vi "Sinc generator to TDMS.vi"() -> ()   [LabVIEW 2025]
uses:
  <vilib>/Analysis/1siggen.llb/Ramp Pattern by Samples.vi
  <vilib>/Analysis/4window.llb/Hamming Window (DBL).vi
  <vilib>/Analysis/2dsp.llb/Real FFT.vi
  <vilib>/Analysis/4window.llb/AllCosWindow (DBL).vi
  <vilib>/Analysis/NI_AALBase.lvlib
  <vilib>/Analysis/NI_AALPro.lvlib
panel:
  in  "Settings Tabs":T1(tab)
  in  "fc":dbl=567000.0 format="%#_6p"
  in  "Tp":dbl=0.0001 format="%#_6p"
  in  "TBW":dbl=4.0
  in  "Vpk":dbl=0.05 format="%#_6p"
  out "BW":dbl
  out "dt/Ts":dbl
  out "N":dbl
  out "Start":dbl format="%#_6p"
  out "End":dbl format="%#_6p"
  out "fs":dbl format="%#_6p"
  out "RF Size":i32
  out "1/fs":dbl format="%#_6p"
  in  "Delays":T2={"gate_delay"=1e-05, "damping_delay"=5e-06, "initial_delay"=5e-06, "final_delay"=5e-06} {"initial_delay" format="%#_6ps"; "final_delay" format="%#_6ps"; "gate_delay" format="%#_6ps"; "damping_delay" format="%#_6ps"}
  in  "Vhigh":dbl=5.0
  out "Gate Delay Size":i32
  out "Damping Delay Size":i32
  out "Initial Delay Size":i32
  out "Final Delay Size":i32
  in  "Digital Wfm Resampling":enum32{"Same Fs As RF Wfm", "Resampled Fs"}(tab)
  out "Digital Wfm Fs":dbl format="%#_6p"
  out "Digital Wfm dt":dbl format="%#_6p"
  in  "Digital Wfm Resampled Fs":dbl=300000.0 format="%#_6p"
  in  "Wfm Group Name Suffix":string="Wfm1"
  in  "TDMS File Path":path
  in  "Results Tab":T3(tab)
  out "sinc pluse":waveform(dbl)(graph)
  out "carrier":waveform(dbl)(graph)
  out "RF sinc pluse":waveform(dbl)(graph)
  out "RF Pulse Spectrrum Graph":cluster{"Ramp Pattern":dbl[], dbl[]}(graph)
  out "Gate IN":waveform(dbl)(graph)
  out "Damping":waveform(dbl)(graph)
  out "Rx ON":waveform(dbl)(graph)
  out "Modulated RF Signal":waveform(dbl)(graph)
  out "PA ON":waveform(dbl)(graph)
  # "Carrier Frequency fc = 567 kHz\n  - Sampling Frequency fs = 20 x fc\nPluse Duration Tp = 100 us\nTime Bandwidth Product TBW = 4\n  - Bandwidth BW = TBW/Tp\nPeak Amplitude Vpk = 50 mV"
  # "If TDMS File Path specified,\nwill create/replace file"
  # "Example:\nIf Wfm Group Name Suffix = Wfm1, then it creates:\n- FGEN_Wfm1\n    - Chn0\n- DAQ_Wfm1\n    - PA ON\n    - Gate IN\n    - Damping \n    - Rx ON"
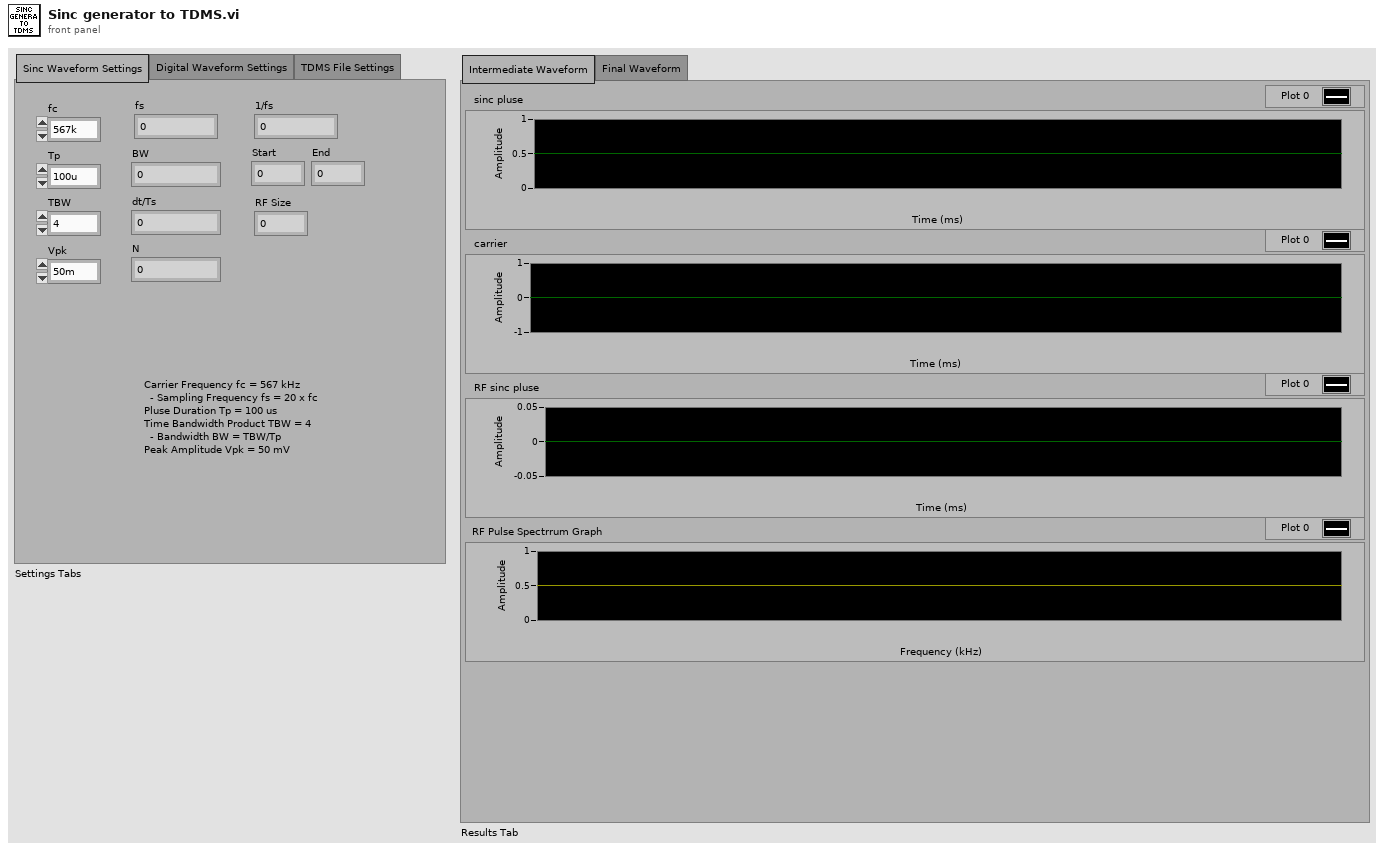
[diagram p1: front panel]
types:
  T1 = enum32{"Sinc Waveform Settings", "Digital Waveform Settings", "TDMS File Settings"}
  T2 = cluster{"gate_delay":dbl, "damping_delay":dbl, "initial_delay":dbl, "final_delay":dbl}
  T3 = enum32{"Intermediate Waveform", "Final Waveform"}
  T4 = enum16{"open", "open or create", "create or replace", "create", "open (read-only)"}
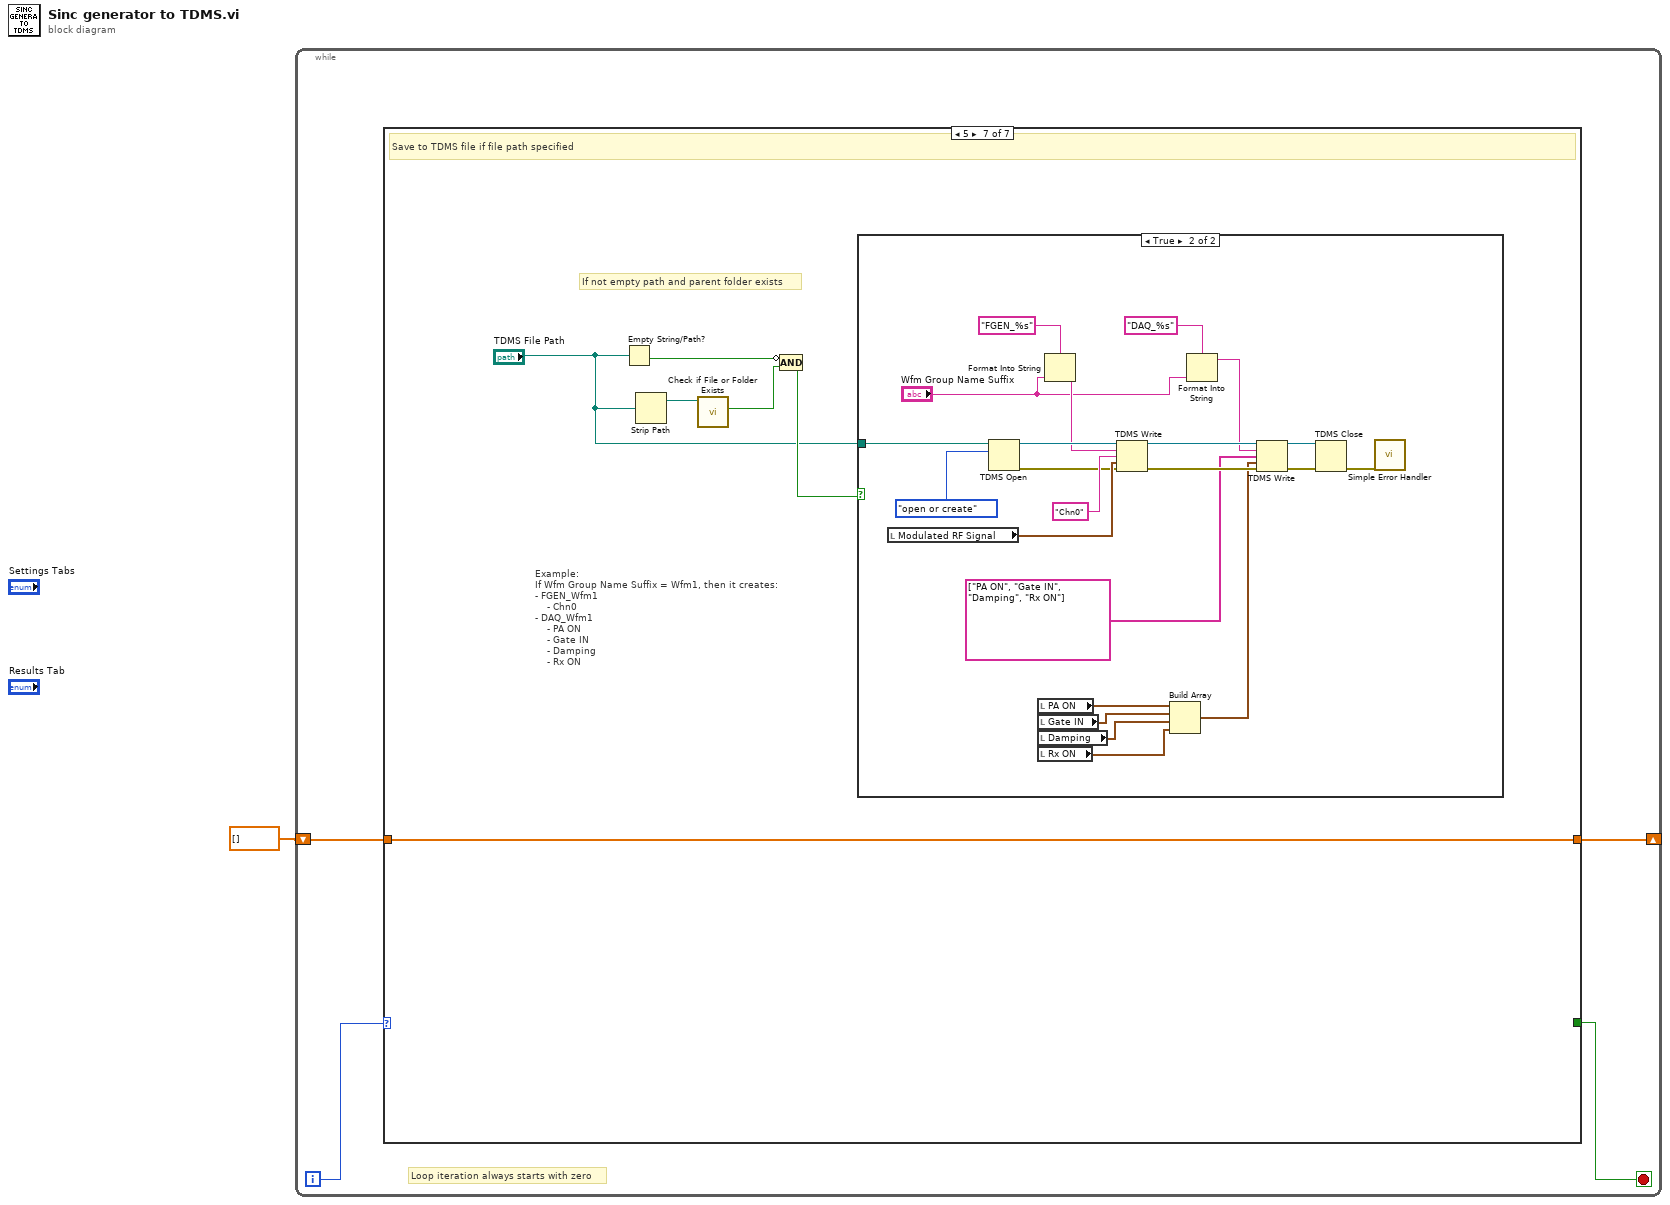
[diagram p0: block diagram]
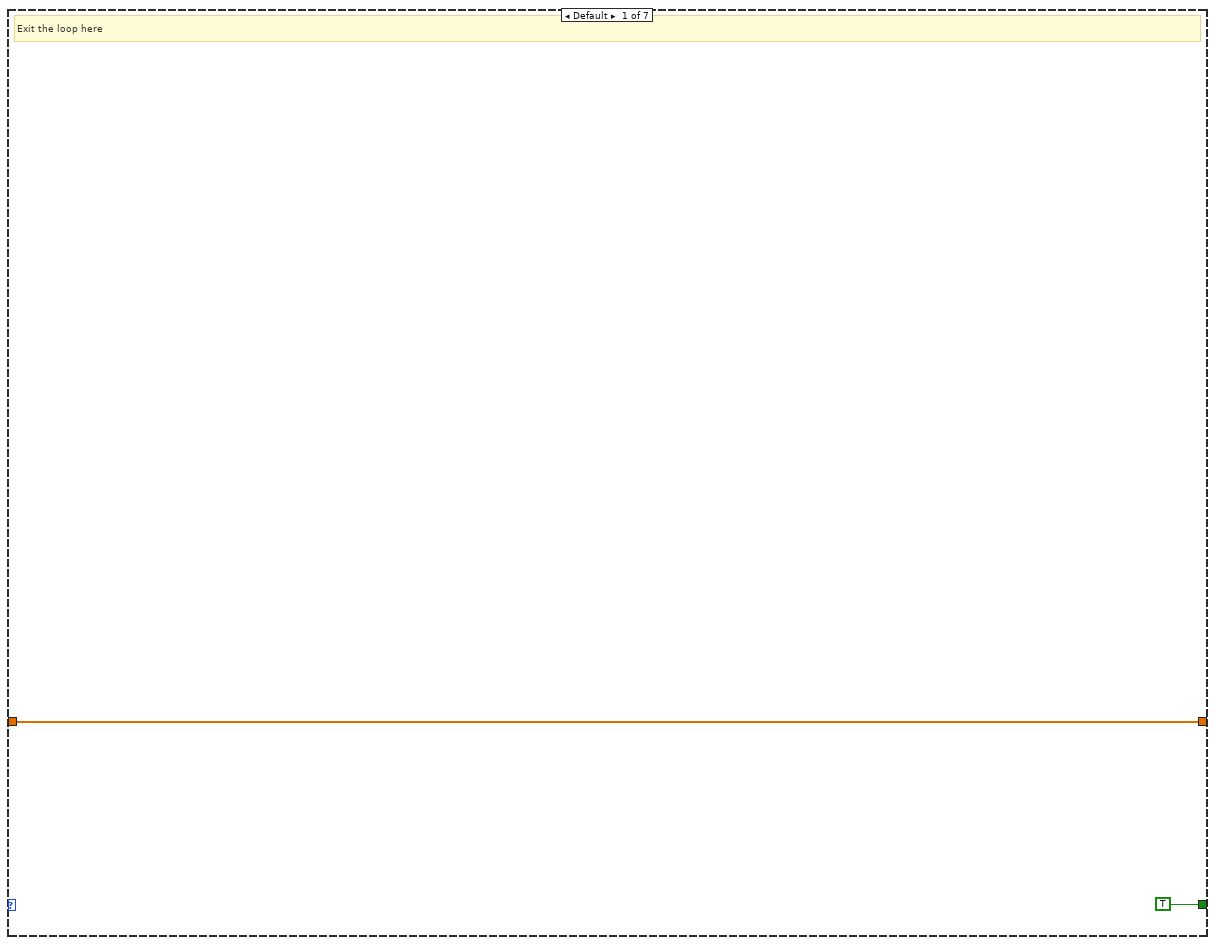
[diagram p2: hidden frame]
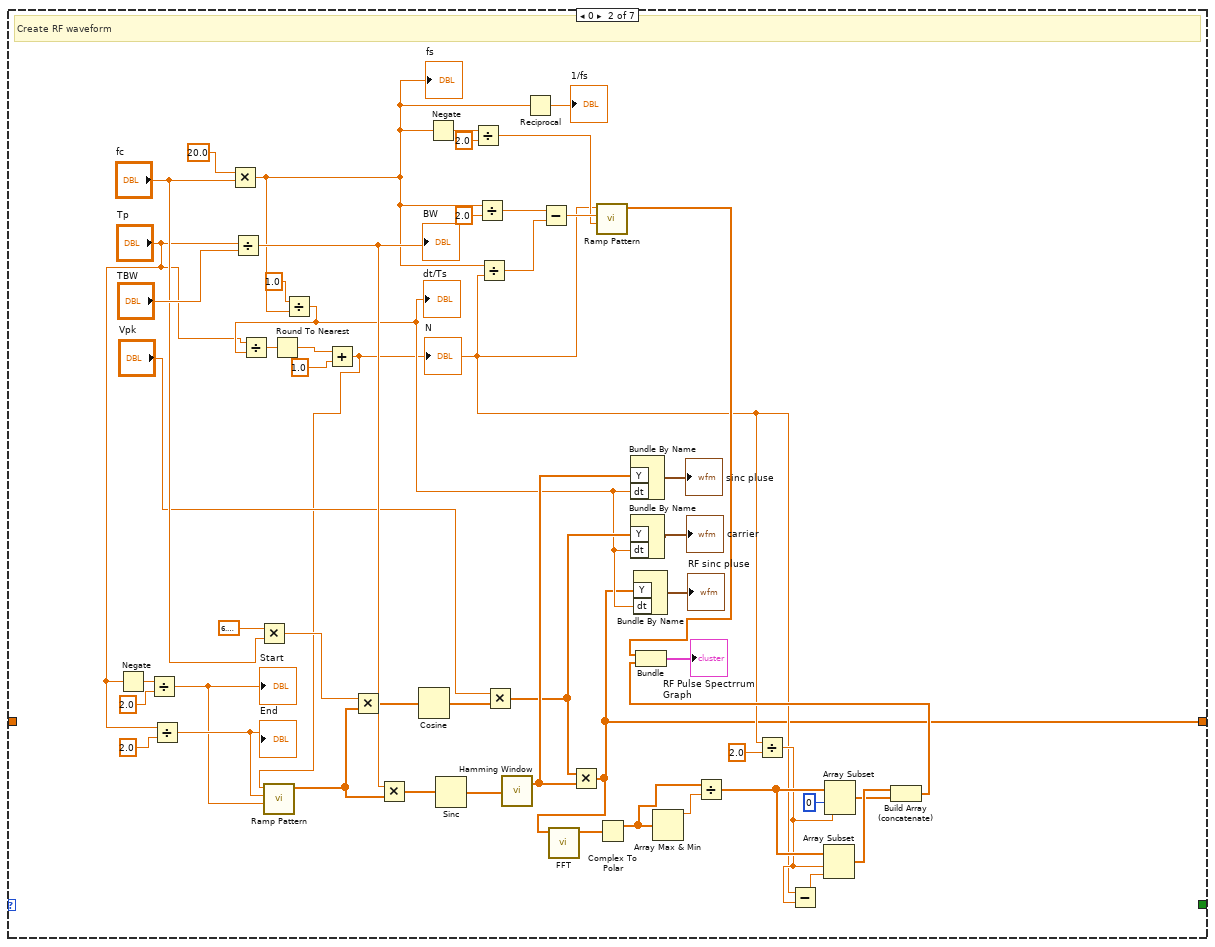
[diagram p3: hidden frame]
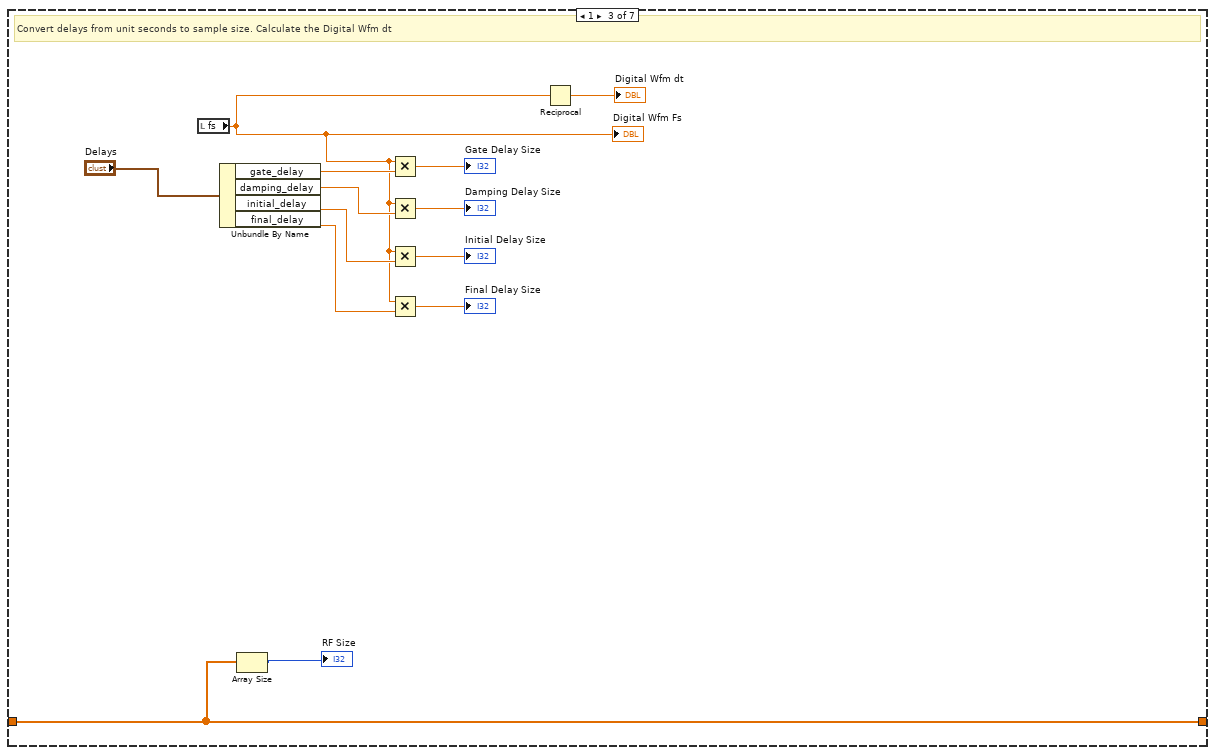
[diagram p4: hidden frame]
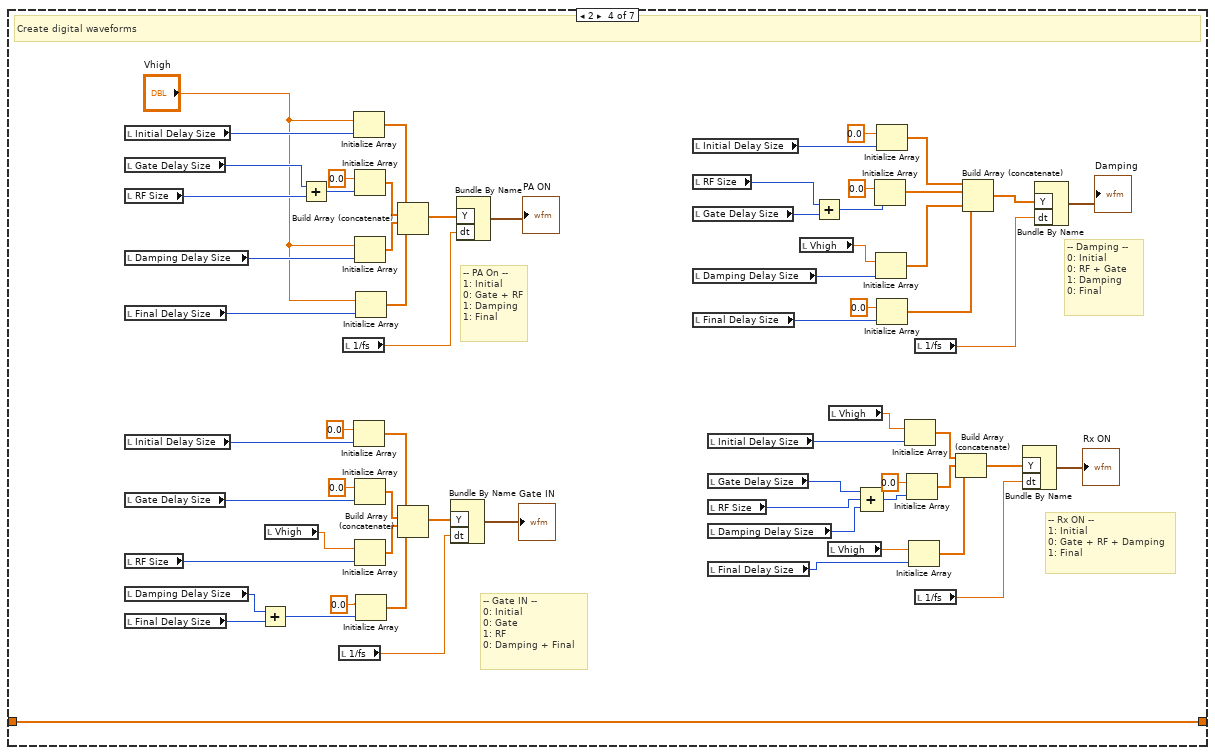
[diagram p5: hidden frame]
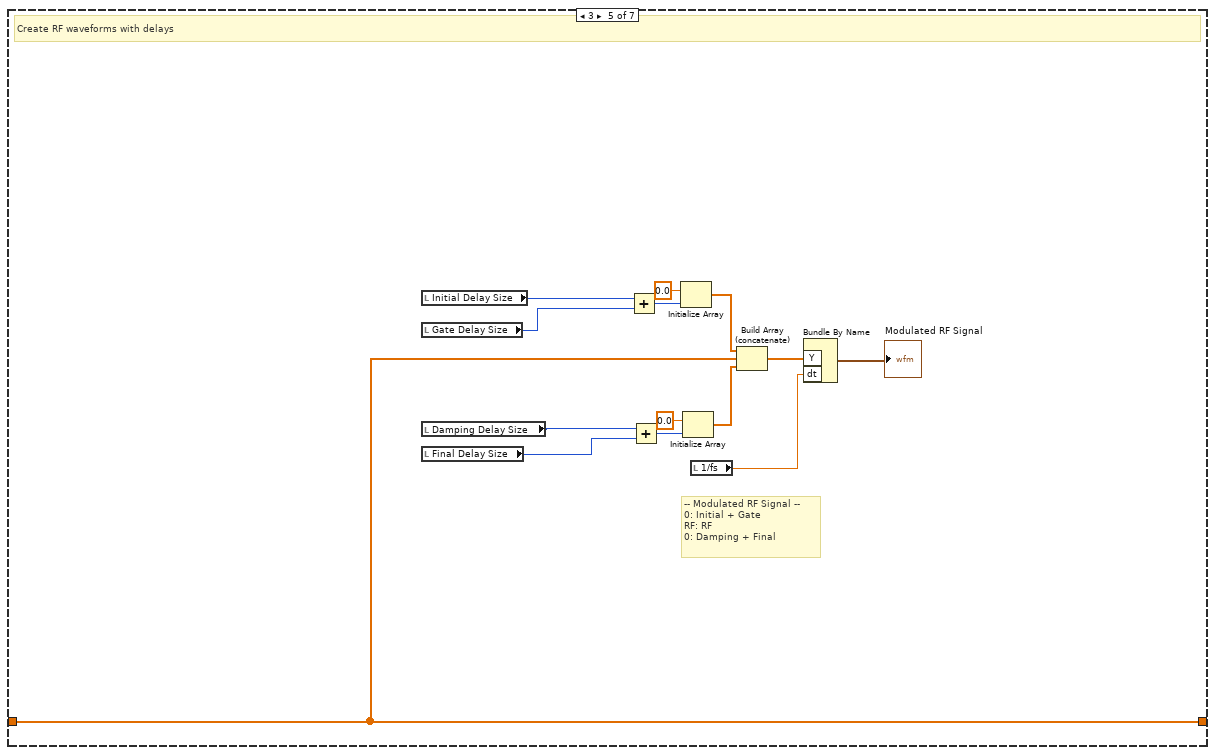
[diagram p6: hidden frame]
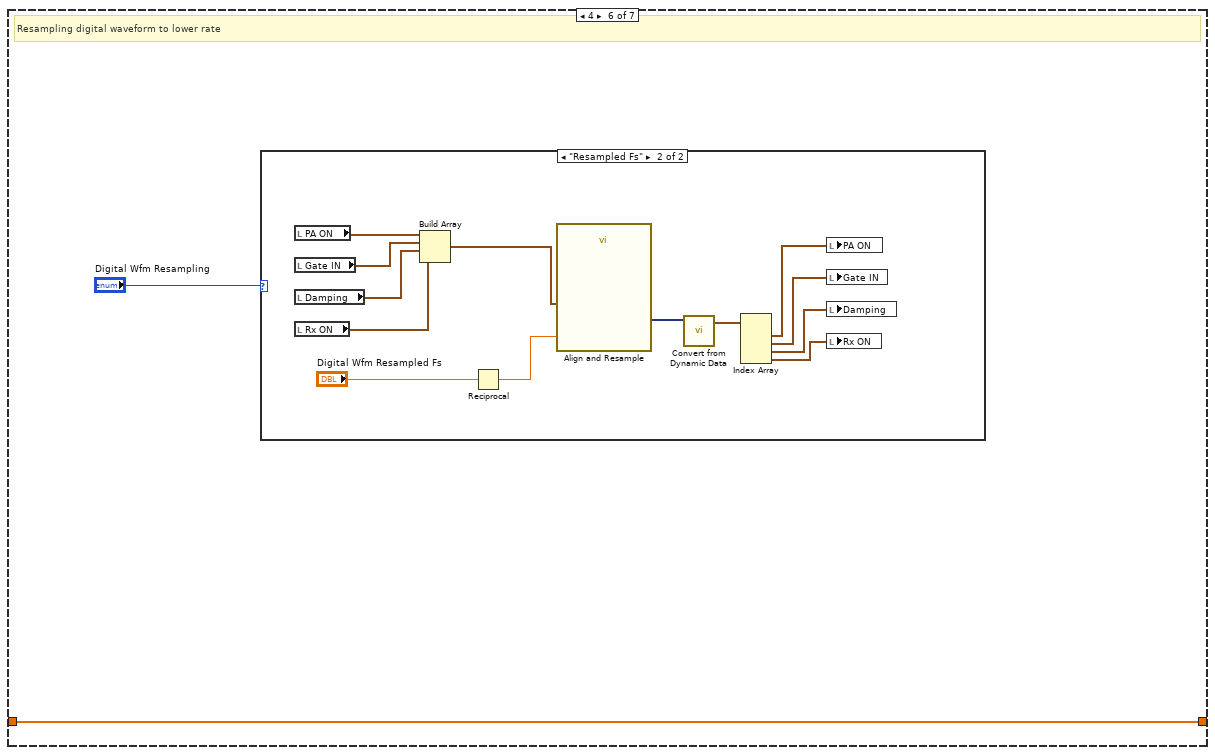
[diagram p7: hidden frame]
diagram:
  n1 = while {
    shift-right: [w4] -> _
    shift-left: dbl[] [] -> [w3]
    i -> [w5]
    stop <- w2 stop-if-true
    # "Loop iteration always starts with zero"
    n2 = case shown="5" w5 {
      tunnel: [TRUE _ _ _ _ _ _] -> w2
      tunnel: [w6 w10 w64 w137 w142 w153 w172] -> w4
      tunnel: w3 -> [w6 _ w64 w137 w142 w153 w172]
      frame Default {
        # "Exit the loop here"
      }
      frame 0 {
        # "Create RF waveform"
        n3 = Negate(x="Tp") -> (-x=w21:dbl)
        n4 = Divide(x=w21, y=2.0) -> (x/y=w32:dbl)
        "Start" <- w32
        n5 = Divide(x="Tp", y=2.0) -> (x/y=w51:dbl)
        "End" <- w51
        n6 = Multiply(x=20.0, y="fc") -> (x*y=w8:dbl)
        "fs" <- w8
        n7 = Divide(x="TBW", y="Tp") -> (x/y=w49:dbl)
        "BW" <- w49
        n8 = Multiply(x=6.283185307179586, y="fc") -> (x*y=w45:dbl)
        n9 = Divide(x=1.0, y=w8) -> (x/y=w22:dbl)
        "dt/Ts" <- w22
        n10 = Divide(x="Tp", y=w22) -> (x/y=w54:dbl)
        n11 = Round To Nearest(number=w54) -> (nearest integer value=w56:dbl)
        n12 = Add(x=w56, y=1.0) -> (x+y=w11:dbl)
        "N" <- w11
        n13 = call-poly <vilib>:"Ramp Pattern.vi"("start"=w32, "end"=w51, "samples"=w11) -> ("Ramp Pattern"=w23:dbl[])  [unwired: 7 in, 1 out]
        n14 = Multiply(x=w45, y=w23) -> (x*y=w44:dbl[])
        n15 = Multiply(x=w49, y=w23) -> (x*y=w50:dbl[])
        n16 = Cosine(x=w44) -> (cos(x)=w42:dbl[])
        n17 = Negate(x=w8) -> (-x=w19:dbl)
        n18 = Sinc(1:w50) -> (0:w48:dbl[])
        n19 = Divide(x=w19, y=2.0) -> (x/y=w13:dbl)
        n20 = Divide(x=w8, y=2.0) -> (x/y=w16:dbl)
        n21 = Divide(x=w8, y=w11) -> (x/y=w15:dbl)
        n22 = Multiply(x="Vpk", y=w42) -> (x*y=w29:dbl[])
        n23 = call-poly <vilib>:"Hamming Window.vi"("X"=w48) -> ("Windowed X"=w31:dbl[])  [unwired: 1 out]
        n24 = Reciprocal(x=w8) -> (1/x=→"1/fs":dbl)
        n25 = Subtract(x=w16, y=w15) -> (x-y=w14:dbl)
        n26 = Multiply(x=w29, y=w31) -> (x*y=w10:dbl[])
        n27 = call-poly <vilib>:"FFT.vi"("X"=w10) -> ("FFT {X}"=w41:cdb[])  [unwired: 9 in, 1 out]
        n28 = call-poly <vilib>:"Ramp Pattern.vi"("start"=w13, "end"=w14, "samples"=w11) -> ("Ramp Pattern"=w12:dbl[])  [unwired: 7 in, 1 out]
        n29 = Complex To Polar(r * e^(i*theta)=w41) -> (r=w25:dbl[])  [unwired: 1 out]
        n30 = Bundle By Name("Y"=w31, "dt"=w22) -> (→"sinc pluse":waveform(dbl))  [unwired: 1 in]
        n31 = Bundle By Name("Y"=w29, "dt"=w22) -> (→"carrier":waveform(dbl))  [unwired: 1 in]
        n32 = Bundle By Name("Y"=w10, "dt"=w22) -> (→"RF sinc pluse":waveform(dbl))  [unwired: 1 in]
        n33 = Array Max & Min(array=w25) -> (max value=w40:dbl)  [unwired: 3 out]
        n34 = Divide(x=w25, y=w40) -> (x/y=w39:dbl[])
        n35 = Divide(x=w11, y=2.0) -> (x/y=w35:dbl)
        n36 = Subtract(x=w11, y=w35) -> (x-y=w36:dbl)
        n37 = Array Subset(array=w39, index=w35, length=w36) -> (w34:dbl[])
        n38 = Array Subset(array=w39, index=0, length=w35) -> (w33:dbl[])
        n39 = Build Array (concatenate)(w34, w33) -> (w24:dbl[])
        n40 = Bundle("Ramp Pattern"=w12, w24) -> (→"RF Pulse Spectrrum Graph":cluster{"Ramp Pattern":dbl[], dbl[]})  [unwired: 1 in]
      }
      frame 1 {
        # "Convert delays from unit seconds to sample size. Calculate the Digital Wfm dt"
        n41 = local read "fs"() -> (w62:dbl)
        "Digital Wfm Fs" <- w62
        n42 = Unbundle By Name("Delays") -> ("gate_delay"=w72:dbl, "damping_delay"=w67:dbl, "initial_delay"=w66:dbl, "final_delay"=w65:dbl)
        n43 = Array Size(array=w64) -> (size(s)=→"RF Size":i32)
        n44 = Multiply(x=w62, y=w72) -> (x*y=→"Gate Delay Size":dbl)
        n45 = Multiply(x=w62, y=w67) -> (x*y=→"Damping Delay Size":dbl)
        n46 = Multiply(x=w62, y=w66) -> (x*y=→"Initial Delay Size":dbl)
        n47 = Multiply(x=w62, y=w65) -> (x*y=→"Final Delay Size":dbl)
        n48 = Reciprocal(x=w62) -> (1/x=→"Digital Wfm dt":dbl)
      }
      frame 2 {
        # "-- Rx ON --\n1: Initial\n0: Gate + RF + Damping\n1: Final"
        # "-- Gate IN --\n0: Initial \n0: Gate \n1: RF\n0: Damping + Final"
        # "-- PA On --\n1: Initial\n0: Gate + RF\n1: Damping\n1: Final"
        # "-- Damping --\n0: Initial\n0: RF + Gate\n1: Damping\n0: Final"
        # "Create digital waveforms"
        n49 = local read "Initial Delay Size"() -> (w93:i32)
        n50 = local read "Gate Delay Size"() -> (w92:i32)
        n51 = local read "RF Size"() -> (w129:i32)
        n52 = local read "Damping Delay Size"() -> (w127:i32)
        n53 = local read "Final Delay Size"() -> (w128:i32)
        n54 = local read "Initial Delay Size"() -> (w124:i32)
        n55 = local read "Gate Delay Size"() -> (w115:i32)
        n56 = local read "RF Size"() -> (w126:i32)
        n57 = local read "Damping Delay Size"() -> (w112:i32)
        n58 = local read "Final Delay Size"() -> (w125:i32)
        n59 = Add(x=w112, y=w125) -> (x+y=w113:i32)
        n60 = local read "Vhigh"() -> (w123:dbl)
        n61 = Add(x=w92, y=w129) -> (x+y=w136:i32)
        n62 = local read "1/fs"() -> (w100:dbl)
        n63 = local read "1/fs"() -> (w101:dbl)
        n64 = Initialize Array("Vhigh", w93) -> (w132:dbl[])
        n65 = Initialize Array(0.0 ("element"), w124) -> (w120:dbl[])
        n66 = Initialize Array(0.0 ("element"), w136) -> (w134:dbl[])
        n67 = Initialize Array("Vhigh", w127) -> (w133:dbl[])
        n68 = Initialize Array(0.0 ("element"), w115) -> (w118:dbl[])
        n69 = Initialize Array(w123, w126) -> (w119:dbl[])
        n70 = Initialize Array("Vhigh", w128) -> (w131:dbl[])
        n71 = Initialize Array(0.0 ("element"), w113) -> (w121:dbl[])
        n72 = Build Array (concatenate)(w132, w134, w133, w131) -> (w130:dbl[])
        n73 = Build Array (concatenate)(w120, w118, w119, w121) -> (w122:dbl[])
        n74 = Bundle By Name("Y"=w122, "dt"=w100) -> (→"Gate IN":waveform(dbl))  [unwired: 1 in]
        n75 = Bundle By Name("Y"=w130, "dt"=w101) -> (→"PA ON":waveform(dbl))  [unwired: 1 in]
        n76 = local read "Initial Delay Size"() -> (w98:i32)
        n77 = local read "RF Size"() -> (w94:i32)
        n78 = local read "Gate Delay Size"() -> (w97:i32)
        n79 = local read "Damping Delay Size"() -> (w96:i32)
        n80 = local read "Final Delay Size"() -> (w95:i32)
        n81 = local read "Initial Delay Size"() -> (w87:i32)
        n82 = local read "Gate Delay Size"() -> (w86:i32)
        n83 = local read "RF Size"() -> (w85:i32)
        n84 = local read "Damping Delay Size"() -> (w84:i32)
        n85 = local read "Final Delay Size"() -> (w83:i32)
        n86 = local read "Vhigh"() -> (w102:dbl)
        n87 = Add(x=w94, y=w97) -> (x+y=w110:i32)
        n88 = local read "Vhigh"() -> (w81:dbl)
        n89 = local read "Vhigh"() -> (w82:dbl)
        n90 = Compound Arithmetic op=ADD(w86, w85, w84) -> (w91:i32)
        n91 = Initialize Array(0.0 ("element"), w110) -> (w108:dbl[])
        n92 = Initialize Array(w102, w96) -> (w107:dbl[])
        n93 = Initialize Array(0.0 ("element"), w98) -> (w106:dbl[])
        n94 = Initialize Array(0.0 ("element"), w95) -> (w104:dbl[])
        n95 = Initialize Array(w82, w87) -> (w79:dbl[])
        n96 = Initialize Array(0.0 ("element"), w91) -> (w89:dbl[])
        n97 = Initialize Array(w81, w83) -> (w80:dbl[])
        n98 = local read "1/fs"() -> (w99:dbl)
        n99 = local read "1/fs"() -> (w73:dbl)
        n100 = Build Array (concatenate)(w79, w89, w80) -> (w88:dbl[])
        n101 = Build Array (concatenate)(w106, w108, w107, w104) -> (w103:dbl[])
        n102 = Bundle By Name("Y"=w88, "dt"=w73) -> (→"Rx ON":waveform(dbl))  [unwired: 1 in]
        n103 = Bundle By Name("Y"=w103, "dt"=w99) -> (→"Damping":waveform(dbl))  [unwired: 1 in]
      }
      frame 3 {
        # "-- Modulated RF Signal --\n0: Initial + Gate\nRF: RF\n0: Damping + Final"
        # "Create RF waveforms with delays"
        n104 = local read "Initial Delay Size"() -> (w143:i32)
        n105 = local read "Gate Delay Size"() -> (w144:i32)
        n106 = local read "Damping Delay Size"() -> (w146:i32)
        n107 = local read "Final Delay Size"() -> (w145:i32)
        n108 = Add(x=w143, y=w144) -> (x+y=w151:i32)
        n109 = Add(x=w146, y=w145) -> (x+y=w149:i32)
        n110 = Initialize Array(0.0 ("element"), w151) -> (w140:dbl[])
        n111 = Initialize Array(0.0 ("element"), w149) -> (w148:dbl[])
        n112 = local read "1/fs"() -> (w138:dbl)
        n113 = Build Array (concatenate)(w140, w142, w148) -> (w147:dbl[])
        n114 = Bundle By Name("Y"=w147, "dt"=w138) -> (→"Modulated RF Signal":waveform(dbl))  [unwired: 1 in]
      }
      frame 4 {
        # "Resampling digital waveform to lower rate"
        n115 = case shown="\"Resampled Fs\"" "Digital Wfm Resampling" {
          frame "Same Fs As RF Wfm", Default {
          }
          frame "Resampled Fs" {
            n116 = local read "PA ON"() -> (w166:waveform(dbl))
            n117 = local read "Gate IN"() -> (w165:waveform(dbl))
            n118 = local read "Damping"() -> (w164:waveform(dbl))
            n119 = local read "Rx ON"() -> (w163:waveform(dbl))
            n120 = Build Array(w166, w165, w164, w163) -> (w162:waveform(dbl)[])
            n121 = Reciprocal(x="Digital Wfm Resampled Fs") -> (1/x=w160:dbl)
            n122 = call "Align and Resample"("dt"=w160, "Signals"=w162) -> ("Resampled Signals"=w159:dynamicdata)  [unwired: 7 in, 2 out]
            n123 = call "Convert from Dynamic Data"("Dynamic Data Type"=w159) -> ("Array of Waveform"=w158:waveform(dbl)[])  [unwired: 3 in]
            n124 = Index Array(array=w158) -> (element #1=w157:waveform(dbl), element #2=w156:waveform(dbl), element #3=w155:waveform(dbl), element #4=w154:waveform(dbl))  [unwired: 4 in]
            n125 = local write "PA ON"(w157) -> ()
            n126 = local write "Gate IN"(w156) -> ()
            n127 = local write "Damping"(w155) -> ()
            n128 = local write "Rx ON"(w154) -> ()
          }
        }
      }
      frame 5 {
        # "Example:\nIf Wfm Group Name Suffix = Wfm1, then it creates:\n- FGEN_Wfm1\n    - Chn0\n- DAQ_Wfm1\n    - PA ON\n    - Gate IN\n    - Damping \n    - Rx ON"
        # "If not empty path and parent folder exists"
        # "Save to TDMS file if file path specified"
        n129 = Empty String/Path?(string/path="TDMS File Path") -> (empty?=w170:bool)
        n130 = Strip Path(path="TDMS File Path") -> (stripped path=w171:path)  [unwired: 1 out]
        n131 = call <vilib>:"Check if File or Folder Exists.vi"("path"=w171) -> ("file or folder exists?"=w169:bool)  [unwired: 8 in, 2 out]
        n132 = Compound Arithmetic op=AND(invert w170, w169) -> (w168:bool)
        n133 = case shown="True" w168 {
          tunnel: "TDMS File Path" -> [_ w194]
          frame False {
          }
          frame True {
            n134 = local read "Modulated RF Signal"() -> (w191:waveform(dbl))
            n135 = TDMS Open(10:T4."open or create" ("operation (0:open)"), 11:w194) -> (0:w185:errorcluster, 3:w192:refnum<k34>)  [unwired: 5 in]
            n136 = local read "PA ON"() -> (w181:waveform(dbl))
            n137 = local read "Gate IN"() -> (w180:waveform(dbl))
            n138 = local read "Damping"() -> (w179:waveform(dbl))
            n139 = local read "Rx ON"() -> (w178:waveform(dbl))
            n140 = Format Into String(format string="FGEN_%s", "Wfm Group Name Suffix") -> (resulting string=w189:string)  [unwired: 2 in, 1 out]
            n141 = TDMS Write(0:w192, 5:w189, 7:"Chn0" ("channel name(s) in (Untitled)"), 9:w191, 11:w185) -> (4:w187:refnum<k34>, 15:w186:errorcluster)  [unwired: 1 in, 2 out]
            n142 = Build Array(w181, w180, w179, w178) -> (w177:waveform(dbl)[])
            n143 = Format Into String(format string="DAQ_%s", "Wfm Group Name Suffix") -> (resulting string=w182:string)  [unwired: 2 in, 1 out]
            n144 = TDMS Write(0:w187, 5:w182, 7:string[] ["PA ON", "Gate IN", "Damping", "Rx ON"] ("channel name(s) in (Untitled)"), 9:w177, 11:w186) -> (4:w174:refnum<k34>, 15:w175:errorcluster)  [unwired: 1 in, 2 out]
            n145 = TDMS Close(8:w175, 11:w174) -> (0:w173:errorcluster)  [unwired: 1 out]
            n146 = call <vilib>:"Simple Error Handler.vi"("error in (no error)"=w173) -> ()  [unwired: 4 in, 5 out]
          }
        }
      }
    }
  }
